vi "TPNT_FindDeviceTP.vi"(8 "error in (no error)":errorcluster, 9 "error":enum16{"none", "on found", "on not found"}(ring), 10 "TP name":string, 11 "Object Refnum In":T5) -> (0 "error out":errorcluster, 1 "index":i32, 2 "TP":T1={"name"="", "type"="", "algor"=[], "update_rate"=0.0, "Limits"={"Alarm Type"="", "Lower "=0.0, "Upper"=0.0, "Nominal"=0.0, "outrange"=FALSE, "Check"=TRUE, "latch"=FALSE, "level"=""}, "Samples"={"samples"=0, "counter"=0, "Values"=[], "Current Value"="", "filter"="", "precision"=2}, "next_update"=0, "Status"="", "monitor"=TRUE, "error"=FALSE, "Log"={"log"=FALSE, "file"=path "", "type"="", "format"="", "updaterate"=0.0, "nex_update"=0, "mode"=""}, "permissions"="", "ID"=""} {"Log"."updaterate" format="%.2f"; "Samples"."Values" format="%.2f"; "Samples"."samples" min=1 step=1; "Limits"."Nominal" format="%.2f"; "Limits"."Upper" format="%.2f"; "Limits"."Lower" format="%.2f"; "update_rate" format="%.2f"}, 3 "Data Refnum out":T5)   [LabVIEW 2016]
uses:
  TPNT_Refnum.ctl
  TPNT_TP.ctl
  TPNT_Limits.ctl
  TPNT_Samples.ctl
  TPNT_Log.ctl
  TPNT_CoreFunction.ctl
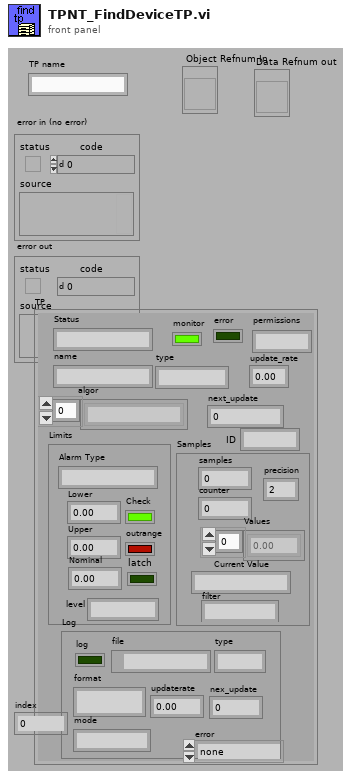
[diagram p1: front panel]
types:
  T1 = typedef "TPNT_TP.ctl" = cluster{"name":string, "type":string, "algor":string[], "update_rate":sgl, "Limits":T2, "Samples":T3, "next_update":u32, "Status":string, "monitor":bool, "error":bool, "Log":T4, "permissions":string, "ID":string}
  T2 = typedef "TPNT_Limits.ctl" = cluster{"Alarm Type":string, "Lower ":dbl, "Upper":dbl, "Nominal":dbl, "outrange":bool, "Check":bool, "latch":bool, "level":string}
  T3 = typedef "TPNT_Samples.ctl" = cluster{"samples":i32, "counter":i32, "Values":dbl[], "Current Value":string, "filter":string, "precision":u8}
  T4 = typedef "TPNT_Log.ctl" = cluster{"log":bool, "file":path, "type":string, "format":string, "updaterate":dbl, "nex_update":u32, "mode":string}
  T5 = typedef "TPNT_Refnum.ctl" = refnum<vi>
  T6 = typedef "TPNT_CoreFunction.ctl" = enum16{"Reset", "Register", "Get Data", "Set Data", "Unregister", "Test", "Get Objects"}
  T7 = typedef "TPNT_DeviceTPs.ctl" = cluster{"device":string, "devupdate":dbl, "next_update":u32, "devinterface":string, "TPs":T1[], "Alarms":bool, "monitor":bool, "log sep":string}
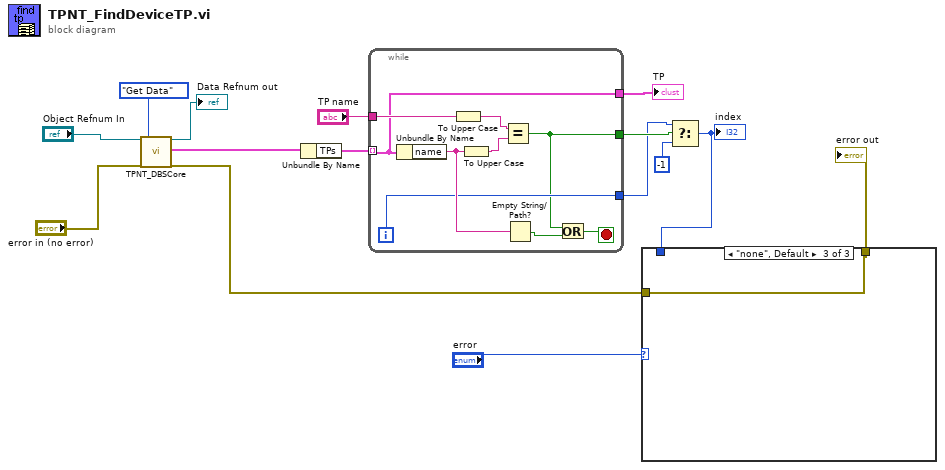
[diagram p0: block diagram]
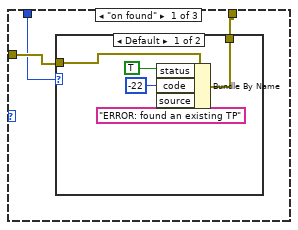
[diagram p2: hidden frame]
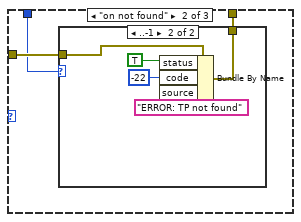
[diagram p4: hidden frame]
diagram:
  n1 = call "TPNT_DBSCore.vi"("Object Refnum In"="Object Refnum In", "error in (no error)"="error in (no error)", "Function (Get Data)"=TPNT_CoreFunction."Get Data") -> ("Object Refnum out"=→"Data Refnum out":T5, "Object Data Out"=w12:T7, "error out"=w5:errorcluster)  [unwired: 2 in, 12 out]
  n2 = Unbundle By Name(w12) -> ("TPs"=w11:T1[])
  n3 = while {
    tunnel: w11 -> [w17] mode=indexing
    tunnel: "TP name" -> [w24]
    tunnel: [w18] -> w8
    tunnel: [w17] -> w6
    tunnel: [w16] -> w9
    i -> [w18]
    stop <- w21 stop-if-true
    n4 = Unbundle By Name(w17) -> ("name"=w20:string)
    n5 = To Upper Case(1:w24) -> (0:w23:string)
    n6 = To Upper Case(1:w20) -> (0:w22:string)
    n7 = Equal?(x=w23, y=w22) -> (x = y?=w16:bool)
    n8 = Empty String/Path?(string/path=w20) -> (empty?=w19:bool)
    n9 = Or(x=w16, y=w19) -> (x .or. y?=w21:bool)
  }
  "TP" <- w6
  n10 = Select(t=w8, s=w9, f=-1) -> (s? t:f=w3:i32)
  "index" <- w3
  n11 = case shown="\"none\", Default" "error" {
    tunnel: w5 -> [w26 w36 w43]
    tunnel: [w27 w35 w43] -> w4
    tunnel: w3 -> [w25 w34 _]
    frame "on found" {
      n12 = case shown="Default" w25 {
        tunnel: [w29 w33] -> w27
        tunnel: w26 -> [w28 w33]
        frame Default {
          n13 = Bundle By Name(cluster=w28, "status"=TRUE, "code"=-22, "source"="ERROR: found an existing TP") -> (w29:errorcluster)
        }
        frame ..-1 {
        }
      }
    }
    frame "on not found" {
      n14 = case shown="..-1" w34 {
        tunnel: [w37 w39] -> w35
        tunnel: w36 -> [w37 w38]
        frame Default {
        }
        frame ..-1 {
          n15 = Bundle By Name(cluster=w38, "status"=TRUE, "code"=-22, "source"="ERROR: TP not found") -> (w39:errorcluster)
        }
      }
    }
    frame "none", Default {
    }
  }
  "error out" <- w4
